vi "more cluster exercise.vi"() -> ()   [LabVIEW 2016]
panel:
  out "Output Cluster":T1 {"Slide" scale=0.0..10.0}
  in  "Input Cluster":T1 {"Slide" scale=0.0..10.0}
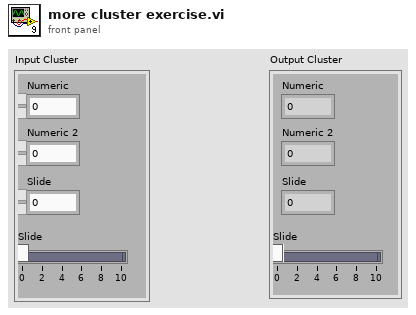
[diagram p1: front panel]
types:
  T1 = cluster{"Numeric":dbl, "Numeric 2":dbl, "Slide":dbl, "Slide":dbl}
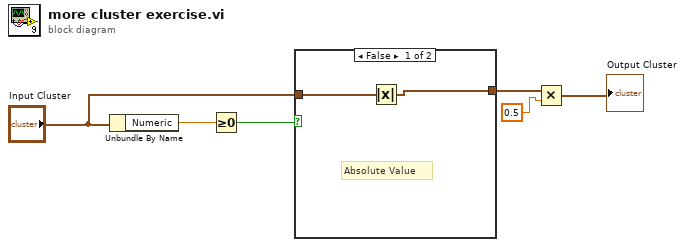
[diagram p0: block diagram]
diagram:
  n1 = Unbundle By Name("Input Cluster") -> ("Numeric"=w6:dbl)
  n2 = Greater Or Equal To 0?(x=w6) -> (x >= 0?=w5:bool)
  n3 = case shown="False" w5 {
    tunnel: "Input Cluster" -> [w8 w9]
    tunnel: [w7 w9] -> w3
    frame False {
      # "Absolute Value"
      n4 = Absolute Value(x=w8) -> (abs(x)=w7:T1)
    }
    frame True {
      # "No change if numeric >=0"
    }
  }
  n5 = Multiply(x=w3, y=0.5) -> (x*y=→"Output Cluster":T1)
